vi "Swerve Drive Striaght SP.vi"(3 "Carry In":bool) -> (1 "Carry out":bool)   [LabVIEW 2016]
uses:
  Robot Global Data.vi
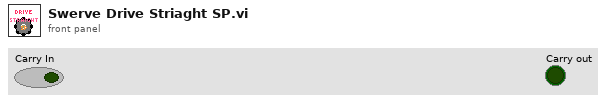
[diagram p1: front panel]
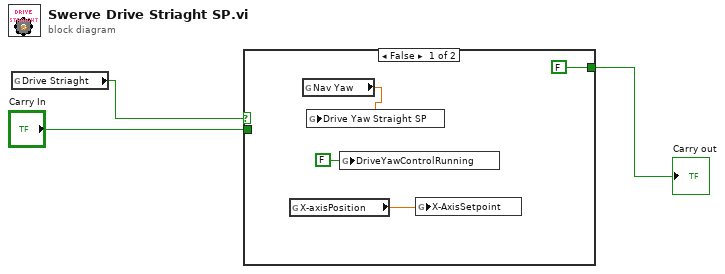
[diagram p0: block diagram]
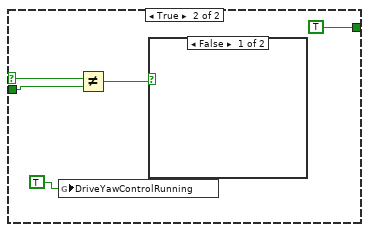
[diagram p2: hidden frame]
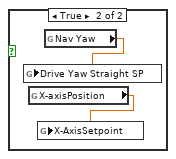
[diagram p3: hidden frame]
diagram:
  n1 = global read "Robot Global Data.vi" "Drive Striaght"() -> (w3:bool)
  n2 = case shown="False" w3 {
    selector: w3 -> [_ w12]
    tunnel: [FALSE TRUE] -> w1
    tunnel: "Carry In" -> [_ w9]
    frame False {
      n3 = global read "Robot Global Data.vi" "X-axisPosition"() -> (w4:dbl)
      n4 = global read "Robot Global Data.vi" "Nav Yaw"() -> (w5:dbl)
      n5 = global write "Robot Global Data.vi" "Drive Yaw Straight SP"(w5) -> ()
      n6 = global write "Robot Global Data.vi" "DriveYawControlRunning"(FALSE ("DriveYawControlRunning")) -> ()
      n7 = global write "Robot Global Data.vi" "X-AxisSetpoint"(w4) -> ()
    }
    frame True {
      n8 = global write "Robot Global Data.vi" "DriveYawControlRunning"(TRUE) -> ()
      n9 = Not Equal?(x=w12, y=w9) -> (x != y?=w11:bool)
      n10 = case shown="False" w11 {
        frame False {
        }
        frame True {
          n11 = global read "Robot Global Data.vi" "X-axisPosition"() -> (w13:dbl)
          n12 = global write "Robot Global Data.vi" "X-AxisSetpoint"(w13) -> ()
          n13 = global read "Robot Global Data.vi" "Nav Yaw"() -> (w14:dbl)
          n14 = global write "Robot Global Data.vi" "Drive Yaw Straight SP"(w14) -> ()
        }
      }
    }
  }
  "Carry out" <- w1
